vi "ponderacionesACZ_ajustes_previos.vi"(6 "id_pon_frecuencia":i32, 7 "last_id_ajuste_previo":string, 8 "error in (no error)":errorcluster, 9 "usuario_registra":i32, 10 "Tabla Referencia Acústica Generador Externo":string[][](table), 11 "BD in":refnum<class "Base de Datos.lvclass">) -> (0 "error out":errorcluster, 3 "BD out":refnum<class "Base de Datos.lvclass">)   [LabVIEW 2019, in "Base de Datos.lvclass"]
uses:
  Base de Datos.lvclass
  Base de Datos.lvclass/Base de Datos.ctl
  SQLiteConnector/SQLiteConnection.lvclass
panel:
  out "Paso 2":string
  # "Tabla que registra los datos de las ponderaciones A,C, Z de Ajustes Previos"
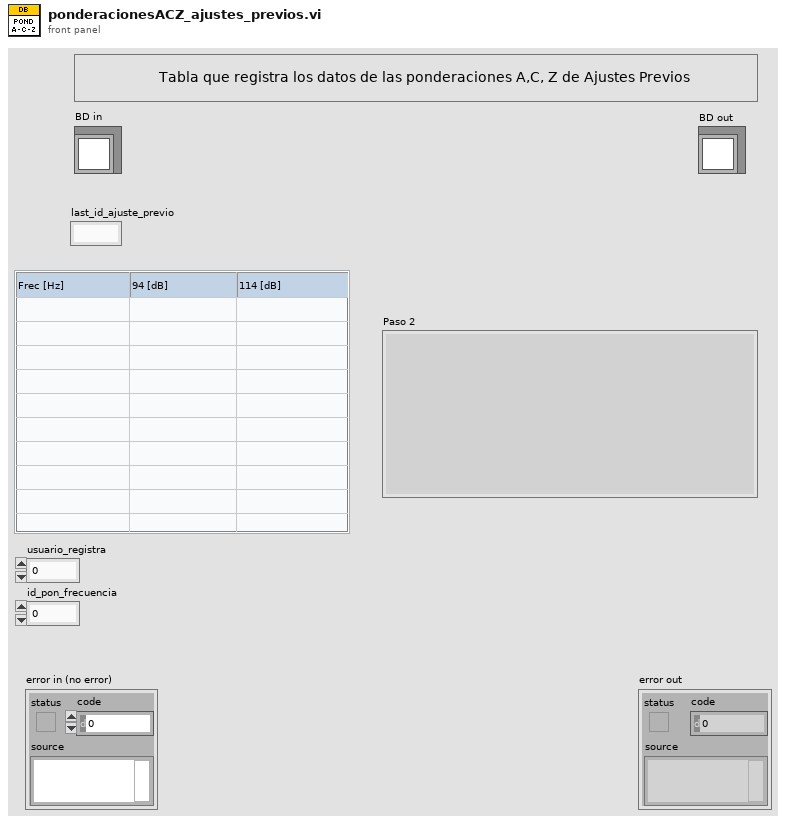
[diagram p1: front panel]
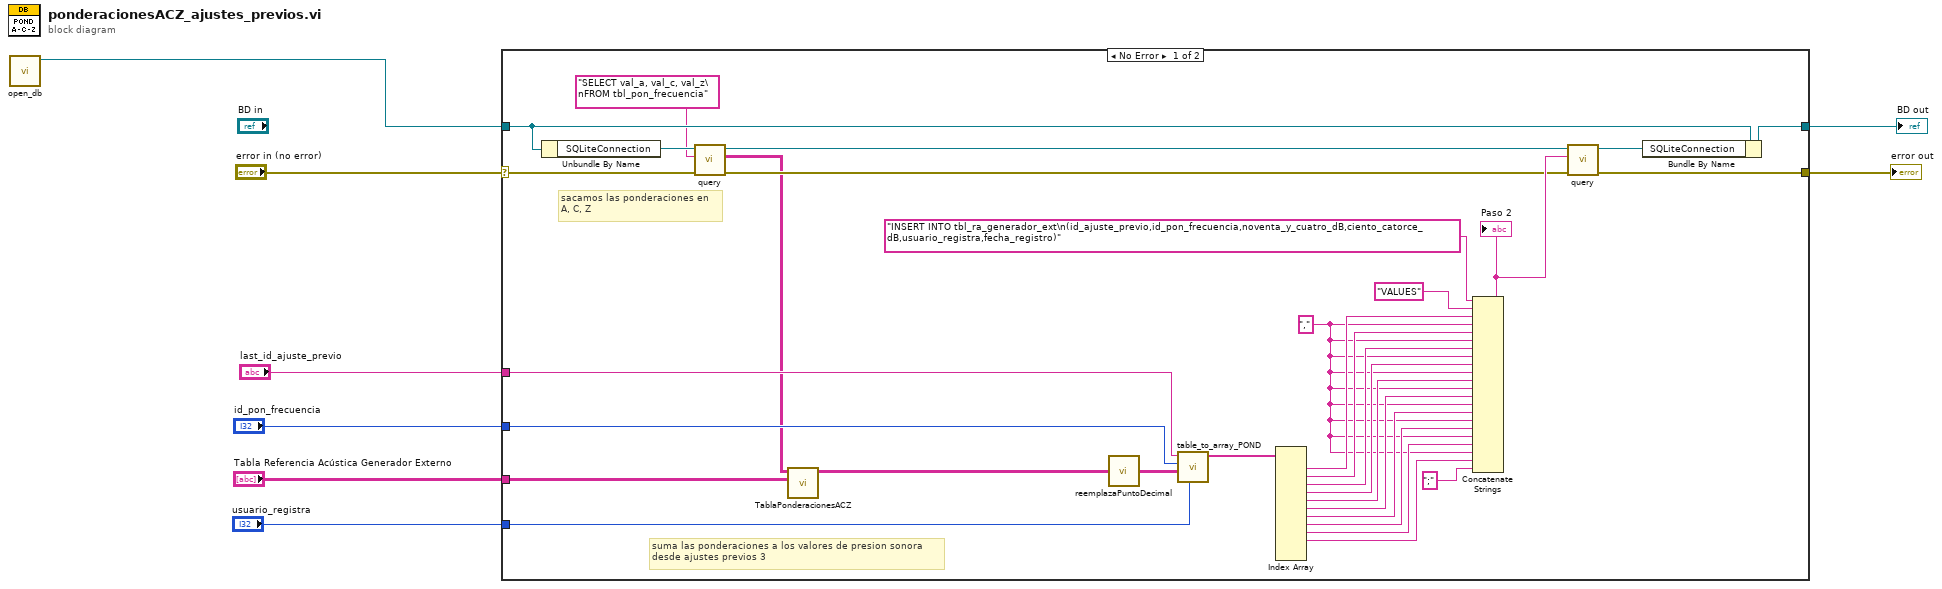
[diagram p0: block diagram]
diagram:
  n1 = call "open_db.vi"() -> ("DB out"=w1:refnum<class "Base de Datos.lvclass">)  [unwired: 10 in, 1 out]
  n2 = case shown="No Error" "error in (no error)" {
    selector: "error in (no error)" -> [w15 w42]
    tunnel: [w40 w42] -> w8
    tunnel: "Tabla Referencia Acústica Generador Externo" -> [w10 _]
    tunnel: "id_pon_frecuencia" -> [w23 _]
    tunnel: "usuario_registra" -> [w22 _]
    tunnel: w1 -> [w16 w41]
    tunnel: "last_id_ajuste_previo" -> [w21 _]
    tunnel: [w20 w41] -> w2
    frame No Error {
      w27 = "," ("string")
      # "suma las ponderaciones a los valores de presion sonora\ndesde ajustes previos 3"
      # "sacamos las ponderaciones en\nA, C, Z"
      n3 = Unbundle By Name(w16) -> ("SQLiteConnection"=w17:refnum<class "SQLiteConnection.lvclass">)
      n4 = call "query.vi"("error in (no error)"=w15, "SQL Statement"="SELECT val_a, val_c, val_z\nFROM tbl_pon_frecuencia" ("format string"), "object in"=w17) -> ("error out"=w14:errorcluster, "result"=w11:string[][], "object out"=w13:refnum<class "SQLiteConnection.lvclass">)  [unwired: 5 in, 1 out]
      n5 = call "TablaPonderacionesACZ.vi"("Tabla Referencia Acústica Generador Externo"=w10, "PonderacionesACZ"=w11) -> ("TablaPonderaciones"=w9:string[][])  [unwired: 9 in]
      n6 = call "reemplazaPuntoDecimal.vi"("Tabla Referencia Acústica Generador Externo in"=w9) -> ("Tabla Referencia Acústica Generador Externo out"=w18:string[][])
      n7 = call "table_to_array_POND.vi"("usuario_registra"=w22, "Tabla Referencia Acústica Generador Externo"=w18, "id_pon_frecuencia"=w23, "last_id_ajuste_previo"=w21) -> ("Array"=w37:string[])  [unwired: 6 in, 1 out]
      n8 = Index Array(array=w37) -> (element #1=w36:string, element #2=w35:string, element #3=w34:string, element #4=w33:string, element #5=w32:string, element #6=w31:string, element #7=w30:string, element #8=w29:string, element #9=w28:string, element #10=w26:string)  [unwired: 12 in, 2 out]
      n9 = Concatenate Strings("INSERT INTO tbl_ra_generador_ext\n(id_ajuste_previo,id_pon_frecuencia,noventa_y_cuatro_dB,ciento_catorce_dB,usuario_registra,fecha_registro)" ("format string"), "VALUES" ("string"), w36, w27, w35, w27, w34, w27, w33, w27, w32, w27, w31, w27, w30, w27, w29, w27, w28, w27, w26, ";" ("string")) -> (w24:string)
      "Paso 2" <- w24
      n10 = call "query.vi"("error in (no error)"=w14, "SQL Statement"=w24, "object in"=w13) -> ("error out"=w40:errorcluster, "object out"=w19:refnum<class "SQLiteConnection.lvclass">)  [unwired: 5 in, 2 out]
      n11 = Bundle By Name(cluster=w16, "SQLiteConnection"=w19) -> (w20:refnum<class "Base de Datos.lvclass">)
    }
    frame Error {
    }
  }
  "error out" <- w8
  "BD out" <- w2
